vi "LVOBJ Get.vi"(8 "error in (no error)":errorcluster, 9 "Default":T1, 10 "JSON Path":string[](array[string]), 11 "Element in":T1) -> (0 "error out":errorcluster, 1 "Value":T1, 2 "Exists?":bool, 3 "Element out":T1)   [LabVIEW 2019, in "labview_json.lvlib"]
uses:
  labview_json.lvlib
  Value.ctl
  Value Type.ctl
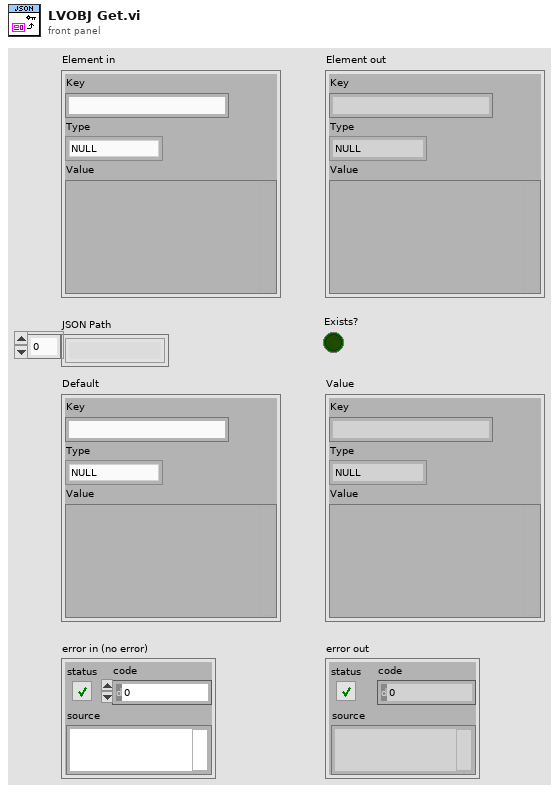
[diagram p1: front panel]
types:
  T1 = typedef "labview_json.lvlib/Value.ctl" = cluster{"Key":string, "Type":T2, "Value":variant}
  T2 = typedef "labview_json.lvlib/Value Type.ctl" = enum8{"NULL", "OBJECT", "ARRAY", "BOOL", "INT", "UINT", "FLOAT", "STRING"}
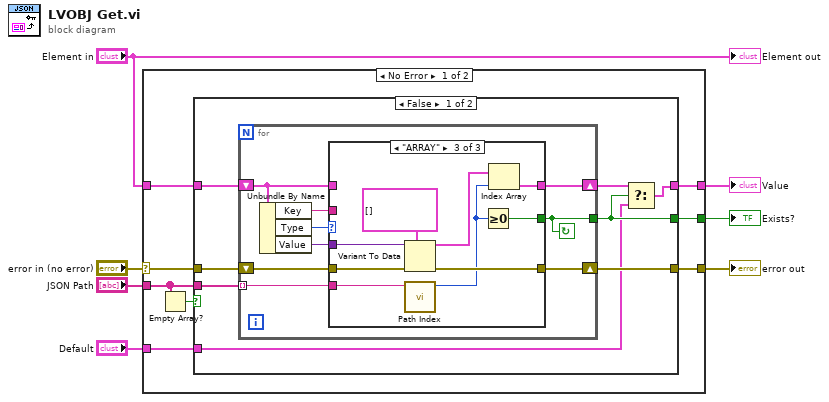
[diagram p0: block diagram]
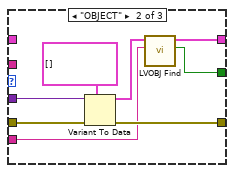
[diagram p3: hidden frame]
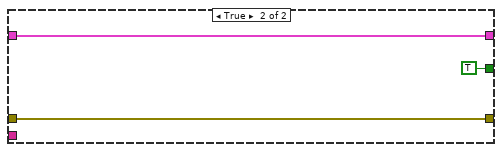
[diagram p4: hidden frame]
diagram:
  n1 = case shown="No Error" "error in (no error)" {
    selector: "error in (no error)" -> [w15 w56]
    tunnel: "JSON Path" -> [w9 _]
    tunnel: [w14 w56] -> w5
    tunnel: [w10 w55] -> w4
    tunnel: "Default" -> [w11 w55]
    tunnel: "Element in" -> [w13 _]
    tunnel: [w12 _] -> w2
    frame No Error {
      n2 = Empty Array?(array=w9) -> (empty?=w8:bool)
      n3 = case shown="False" w8 {
        tunnel: w9 -> [w23 _]
        tunnel: w15 -> [w22 w52]
        tunnel: [w21 w52] -> w14
        tunnel: w13 -> [w20 w54]
        tunnel: [w19 TRUE] -> w12
        tunnel: w11 -> [w18 _]
        tunnel: [w16 w54] -> w10
        frame False {
          n4 = for {
            tunnel: w23 -> [w29] mode=indexing
            shift-right: [w27] -> w21
            shift-left: w22 -> [w28]
            shift-right: [w26] -> w17
            shift-left: w20 -> [w25]
            tunnel: [w24] -> w19
            stop <- w24 continue-if-true
            n5 = Unbundle By Name(w25) -> ("Key"=w30:string, "Type"=w32:T2, "Value"=w31:variant)
            n6 = case shown="\"ARRAY\"" w32 {
              tunnel: w31 -> [_ w42 w51]
              tunnel: w30 -> [_ _ _]
              tunnel: w29 -> [_ w35 w44]
              tunnel: w28 -> [w34 w40 w49]
              tunnel: [w34 w39 w48] -> w27
              tunnel: [w33 w37 w46] -> w26
              tunnel: w25 -> [w33 _ _]
              tunnel: [_ w36 w45] -> w24
              frame Default {
              }
              frame "OBJECT" {
                n7 = Variant To Data(error in=w40, type=T1[] [] ("Values"), Variant=w42) -> (data=w38:T1[], error out=w39:errorcluster)
                n8 = call "LVOBJ Find.vi"("Key"=w35, "Values"=w38) -> ("Found?"=w36:bool, "Value"=w37:T1)  [unwired: 8 in]
              }
              frame "ARRAY" {
                n9 = Variant To Data(error in=w49, type=T1[] [] ("Values"), Variant=w51) -> (data=w47:T1[], error out=w48:errorcluster)
                n10 = call "Path Index.vi"("JSON Path"=w44) -> ("Index"=w43:i32)  [unwired: 10 in]
                n11 = Greater Or Equal To 0?(x=w43) -> (x >= 0?=w45:bool)
                n12 = Index Array(array=w47, index=w43) -> (element=w46:T1)
              }
            }
          }
          n13 = Select(t=w17, s=w19, f=w18) -> (s? t:f=w16:T1)
        }
        frame True {
        }
      }
    }
    frame Error {
    }
  }
  "error out" <- w5
  "Value" <- w4
  "Exists?" <- w2
  "Element out" <- "Element in"
